vi "ZplaneSearch.vi"(8 "error in (no error)":errorcluster, 9 "POI":i32[](array[numeric]), 10 "ImageArray":T1[](array[typedef])) -> (0 "error out":errorcluster, 2 "ZplaneIndex":i32)   [LabVIEW 2020]
uses:
  <vilib>/vision/Image Controls.llb/IMAQ Image.ctl
  <vilib>/vision/NI_Vision_Development_Module.lvlib
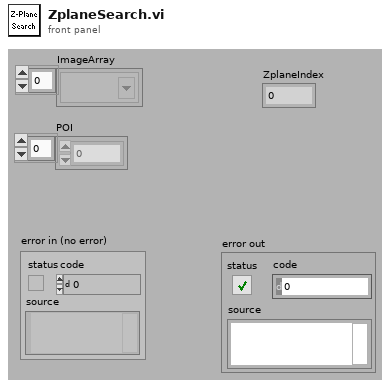
[diagram p1: front panel]
types:
  T1 = typedef "IMAQ Image.ctl" = refnum<image>
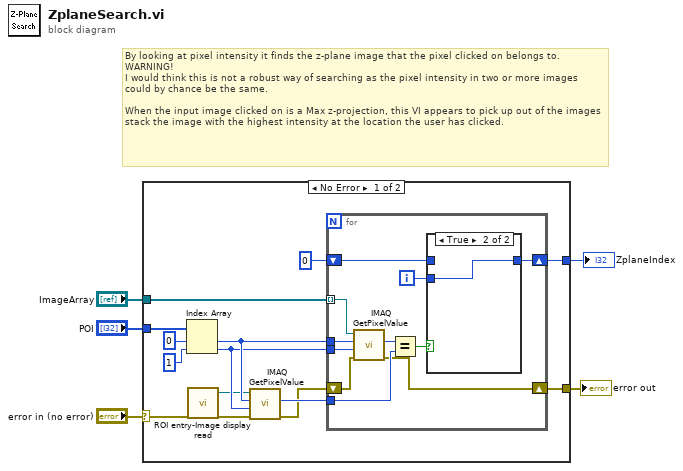
[diagram p0: block diagram]
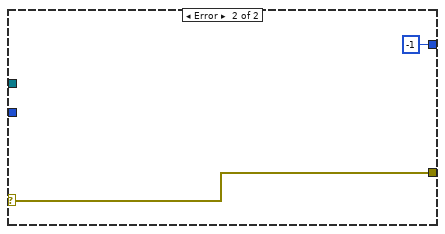
[diagram p3: hidden frame]
diagram:
  # "By looking at pixel intensity it finds the z-plane image that the pixel clicked on belongs to.\nWARNING!\nI would think this is not a robust way of searching as the pixel intensity in two or more images could by chance be the same.\n\nWhen the input image clicked on is a Max z-projection, this VI appears to pick up out of the images stack the image with the highest intensity at the location the user has clicked."
  n1 = case shown="No Error" "error in (no error)" {
    selector: "error in (no error)" -> [w8 w33]
    tunnel: "ImageArray" -> [w18 _]
    tunnel: "POI" -> [w15 _]
    tunnel: [w9 w33] -> w3
    tunnel: [w6 -1] -> w1
    frame No Error {
      n2 = Index Array(array=w15, index #1=0 ("index"), index #2=1 ("index")) -> (element #1=w14:i32, element #2=w13:i32)
      n3 = call "ROI entry-Image display read.vi"() -> ("CurrentImage"=w11:T1)  [unwired: 4 in, 1 out]
      n4 = call "IMAQ GetPixelValue"("Image"=w11, "X Coordinate"=w14, "Y Coordinate"=w13, "error in (no error)"=w8) -> ("Pixel Value (I16)"=w12:i16, "error out"=w10:errorcluster)  [unwired: 2 in, 3 out]
      n5 = for {
        tunnel: w18 -> [w29] mode=indexing
        tunnel: w14 -> [w27]
        tunnel: w13 -> [w26]
        tunnel: w12 -> [w25]
        shift-right: [w22] -> w9
        shift-left: w10 -> [w21]
        shift-right: [w19] -> w6
        shift-left: 0 -> [w20]
        i -> [w23]
        n6 = call "IMAQ GetPixelValue"("Image"=w29, "X Coordinate"=w27, "Y Coordinate"=w26, "error in (no error)"=w21) -> ("Pixel Value (I16)"=w28:i16, "error out"=w22:errorcluster)  [unwired: 2 in, 3 out]
        n7 = Equal?(x=w28, y=w25) -> (x = y?=w24:bool)
        n8 = case shown="True" w24 {
          tunnel: w23 -> [_ w31]
          tunnel: w20 -> [w30 _]
          tunnel: [w30 w31] -> w19
          frame False {
          }
          frame True {
          }
        }
      }
    }
    frame Error {
    }
  }
  "error out" <- w3
  "ZplaneIndex" <- w1
